vi "ConvertStringToScanList.vi"(11 "String":string) -> (3 "Scan List":string)   [LabVIEW 2012, in "Keithley-7001.lvlib"]
uses:
  Keithley-7001.lvlib
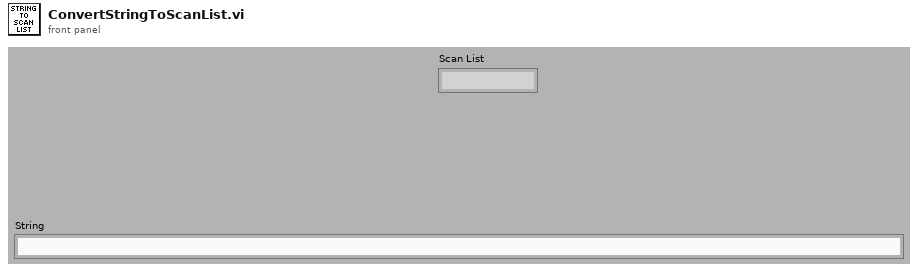
[diagram p1: front panel]
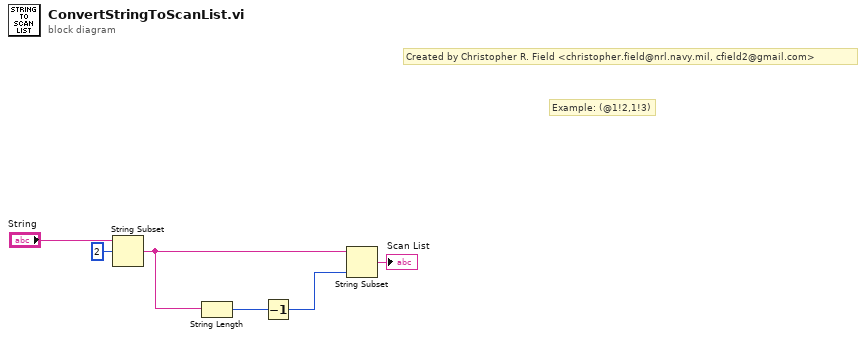
[diagram p0: block diagram]
diagram:
  # "Created by Christopher R. Field <christopher.field@nrl.navy.mil, cfield2@gmail.com>"
  # "Example: (@1!2,1!3)"
  n1 = String Subset(string="String", offset (0)=2) -> (substring=w3:string)  [unwired: 1 in]
  n2 = String Length(string=w3) -> (length=w4:i32)
  n3 = Decrement(x=w4) -> (x-1=w2:i32)
  n4 = String Subset(string=w3, length (rest)=w2) -> (substring=→"Scan List":string)  [unwired: 1 in]
